vi "Set Interface Type.vi"(8 "error in (no error)":errorcluster, 10 "Mode":enum16{"LOCAL", "REMOTE", "LOCKOUT"}(ring), 11 "N5745A in":refnum<class "5745A.lvclass">) -> (0 "error out":errorcluster, 3 "N5745A out":refnum<class "5745A.lvclass">)   [LabVIEW 2018, in "5745A.lvlib" / "5745A.lvclass"]
doc: "This method is used to set the N5745A instrument's operation from its front Button/Knobs (0), LAN/USB/GPIB with read-only at front display (1), LAN/USB/GPIB with disabled front Buttons/Knobs."
uses:
  5745A.lvclass
  builds/Power_Supply.lvlibp/Power Supply.lvclass
  C:/Users/Ron.Dexter.LUMINARTECH/Desktop/builds/Power_Supply.lvlibp/Power Supply.lvclass
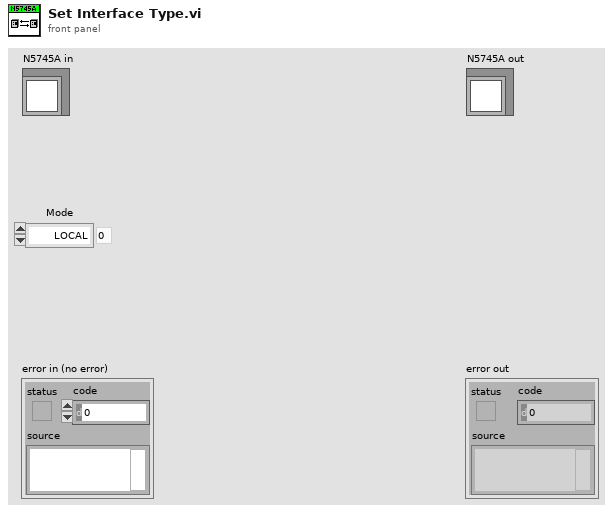
[diagram p1: front panel]
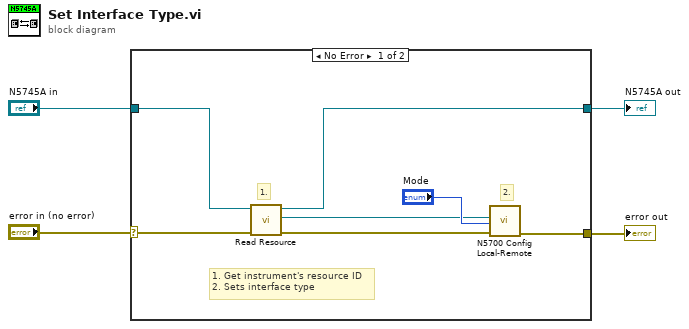
[diagram p0: block diagram]
diagram:
  n1 = case shown="No Error" "error in (no error)" {
    selector: "error in (no error)" -> [w11 w13]
    tunnel: [w7 w13] -> w3
    tunnel: [w5 w12] -> w1
    tunnel: "N5745A in" -> [w6 w12]
    frame No Error {
      # "1. Get instrument's resource ID\n2. Sets interface type"
      # "2."
      # "1."
      n2 = call "Read Resource.vi"("error in"=w11, "Power Supply in"=w6) -> ("error out"=w9:errorcluster, "Resource"=w8:refnum<visa-resource-name>, "Power Supply out"=w5:refnum<class "5745A.lvclass">)  [unwired: 7 in]
      n3 = call <instrlib>:"N5700 Config Local-Remote.vi"("error"=w9, "Mode"="Mode", "VISA"=w8) -> ("error out"=w7:errorcluster)  [unwired: 4 in, 1 out]
    }
    frame Error {
    }
  }
  "error out" <- w3
  "N5745A out" <- w1
